vi "Webcam AE_old.vi"(8 "error in (no error)":errorcluster, 11 "Camera States":enum16{"EXIT", "ACQ", "INIT"}(ring)=enum."INIT") -> (0 "error out":errorcluster, 3 "Image":T1(plugin-control))   [LabVIEW 2018]
uses:
  <vilib>/userdefined/High Color/IMAQdx.ctl
  <vilib>/vision/driver/NI_Vision_Acquisition_Software.lvlib
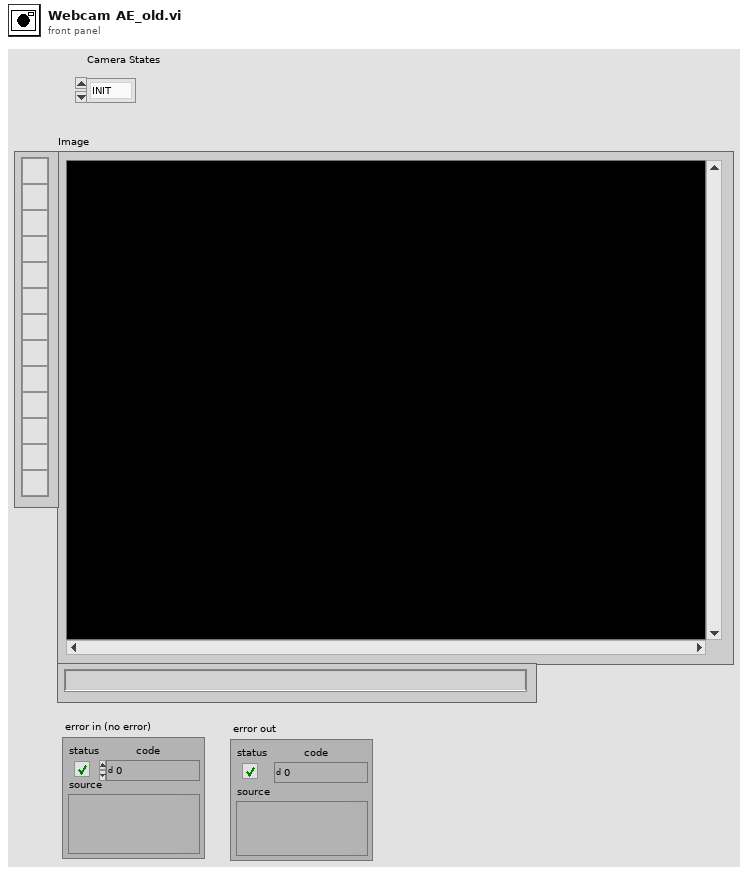
[diagram p1: front panel]
types:
  T1 = typedef "IMAQ Image.ctl" = refnum<image>
  T2 = typedef "IMAQdx.ctl" = refnum<k21>
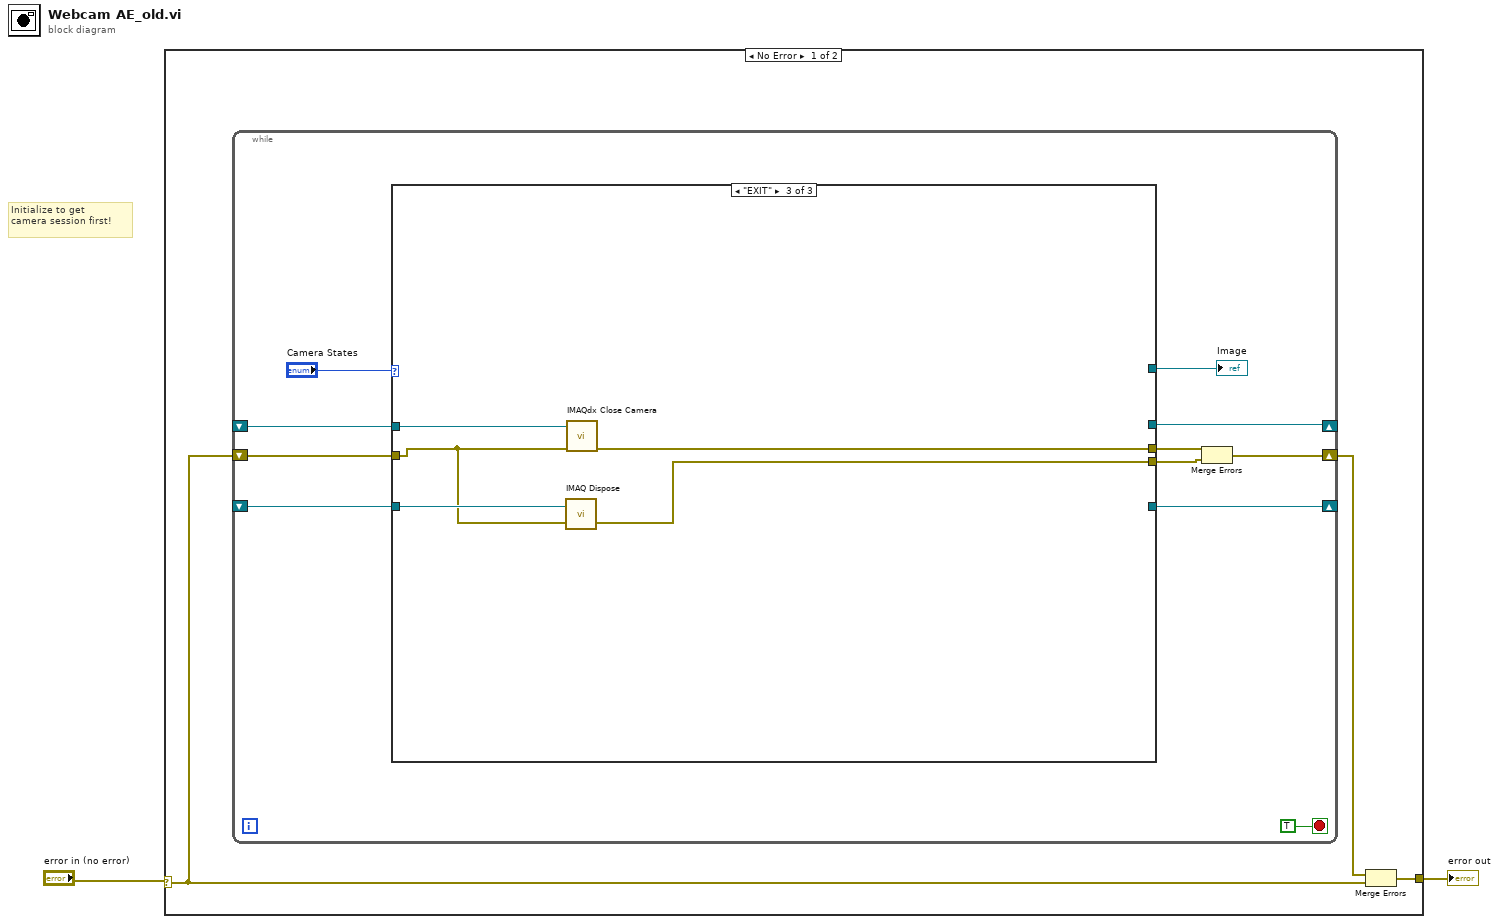
[diagram p0: block diagram]
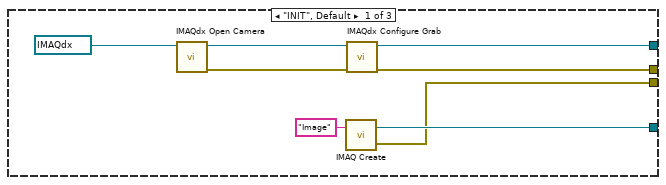
[diagram p2: hidden frame]
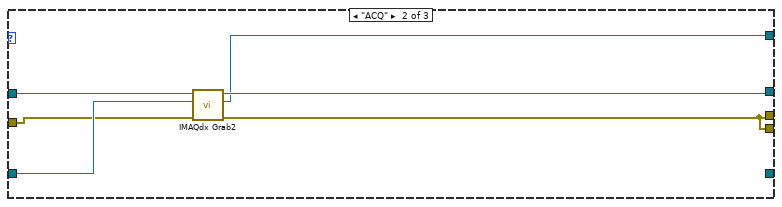
[diagram p3: hidden frame]
diagram:
  # "Initialize to get \ncamera session first!"
  n1 = case shown="No Error" "error in (no error)" {
    selector: "error in (no error)" -> [w3 w36]
    tunnel: [w5 w36] -> w1
    frame No Error {
      n2 = while {
        shift-right: [w15] -> _
        shift-left: _ -> [w10]
        shift-right: [w11] -> w4
        shift-left: w3 -> [w9]
        shift-right: [w14] -> _
        shift-left: _ -> [w8]
        stop <- TRUE stop-if-true
        n3 = case shown="\"EXIT\"" "Camera States" {
          tunnel: [w21 w27 _] -> w15
          tunnel: [w20 w26 w32] -> w13
          tunnel: [w18 _ _] -> w14
          tunnel: [w17 w26 w31] -> w12
          tunnel: w10 -> [_ w30 w35]
          tunnel: w9 -> [_ w28 w33]
          tunnel: w8 -> [_ w29 w34]
          tunnel: [_ w25 _] -> w6
          frame "INIT", Default {
            n4 = call <vilib>:"IMAQdx Open Camera.vi"("Session In"=T2 "cam1") -> ("error out"=w23:errorcluster, "Session Out"=w24:T2)  [unwired: 9 in]
            n5 = call "IMAQ Create"("Image Name"="Image") -> ("New Image"=w18:T1, "error out"=w17:errorcluster)  [unwired: 4 in]
            n6 = call <vilib>:"IMAQdx Configure Grab.vi"("error in"=w23, "Session In"=w24) -> ("error out"=w20:errorcluster, "Session Out"=w21:T2)  [unwired: 8 in]
          }
          frame "ACQ" {
            n7 = call <vilib>:"IMAQdx Grab2.vi"("error in"=w28, "Image In"=w29, "Session In"=w30) -> ("error out"=w26:errorcluster, "Image Out"=w25:T1, "Session Out"=w27:T2)  [unwired: 5 in, 1 out]
          }
          frame "EXIT" {
            n8 = call "IMAQ Dispose"("Image"=w34, "error in (no error)"=w33) -> ("error out"=w31:errorcluster)  [unwired: 4 in]
            n9 = call <vilib>:"IMAQdx Close Camera.vi"("error in"=w33, "Session In"=w35) -> ("error out"=w32:errorcluster)  [unwired: 9 in]
          }
        }
        "Image" <- w6
        n10 = Merge Errors(w13, w12) -> (w11:errorcluster)
      }
      n11 = Merge Errors(w4, w3) -> (w5:errorcluster)
    }
    frame Error {
    }
  }
  "error out" <- w1
